vi "Master_WriteToDigOut.vi"(8 "error in":errorcluster, 9 "FPGA VI Reference In":refnum<k20>, 10 "Actuators in":T1) -> (0 "error out":errorcluster, 1 "FPGA VI Reference Out":refnum<k20>, 2 "Actuators out":T1)   [LabVIEW 2017]
uses:
  TypeDef_DigitalOuts.ctl
  <vilib>/Utility/error.llb/Error Cluster From Error Code.vi
  <vilib>/rvi/errors/niLvFpgaAdjustHostInterfaceError.vi
  <vilib>/rvi/interface/nirviReadWriteControl/nirviReadWriteControl.xnode
  NiFpgaLv.dll
  <vilib>/rvi/interface/Simulation/niFpgaSimulationCallBeginRW.vi
panel:
  out "Actual out":T1
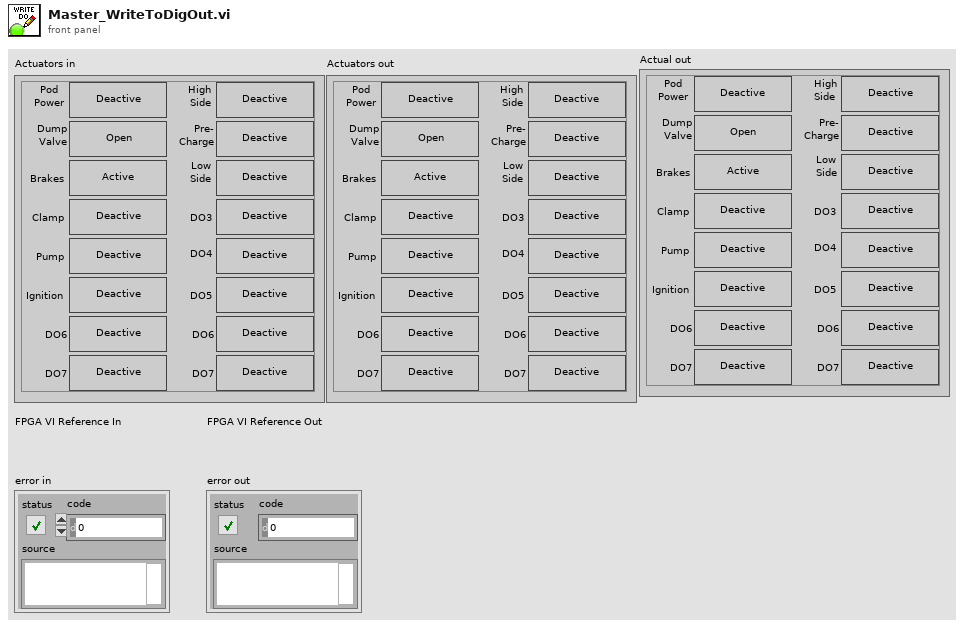
[diagram p1: front panel]
types:
  T1 = typedef "TypeDef_DigitalOuts.ctl" = cluster{"Pod Power":bool, "Dump Valve":bool, "Brakes":bool, "Clamp":bool, "Pump":bool, "Ignition":bool, "DO6":bool, "DO7":bool, "HighSide":bool, "Precharge":bool, "LowSide":bool, "DO3":bool, "DO4":bool, "DO5":bool, "DO62":bool, "DO72":bool}
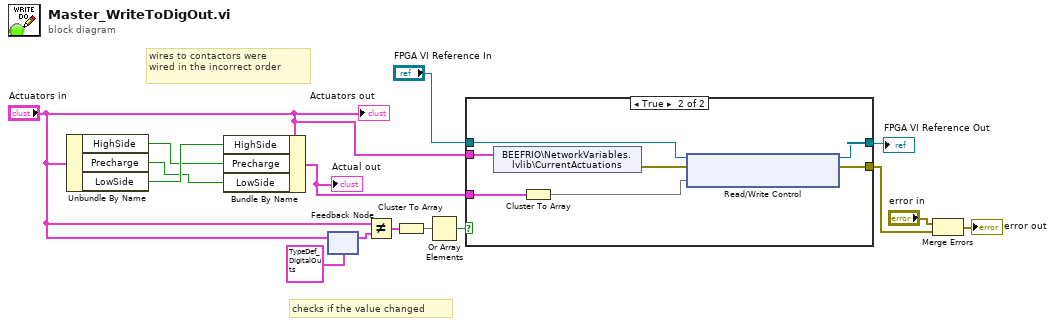
[diagram p0: block diagram]
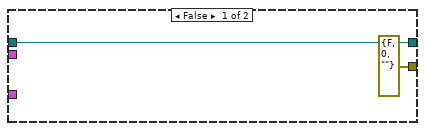
[diagram p2: hidden frame]
diagram:
  # "wires to contactors were\nwired in the incorrect order"
  # "checks if the value changed"
  n1 = Unbundle By Name("Actuators in") -> ("HighSide"=w2:bool, "Precharge"=w1:bool, "LowSide"=w3:bool)
  n2 = Bundle By Name(cluster="Actuators in", "HighSide"=w3, "Precharge"=w2, "LowSide"=w1) -> (w5:T1)
  "Actual out" <- w5
  n3 = feedback-in #1("Actuators in") -> ()
  n4 = feedback #1(T1 {"Pod Power"=FALSE, "Dump Valve"=FALSE, "Brakes"=FALSE, "Clamp"=FALSE, "Pump"=FALSE, "Ignition"=FALSE, "DO6"=FALSE, "DO7"=FALSE, "HighSide"=FALSE, "Precharge"=FALSE, "LowSide"=FALSE, "DO3"=FALSE, "DO4"=FALSE, "DO5"=FALSE, "DO62"=FALSE, "DO72"=FALSE} ("Actuators in")) -> (w15:T1)
  n5 = Not Equal?(x="Actuators in", y=w15) -> (x != y?=w12:T1)
  n6 = Cluster To Array(cluster=w12) -> (array=w11:bool[])
  n7 = Or Array Elements(Boolean array=w11) -> (logical OR=w14:bool)
  n8 = case shown="True" w14 {
    tunnel: [errorcluster {"status"=FALSE, "code"=0, "source"=""} ("error out") w24] -> w7
    tunnel: w5 -> [_ w18]
    tunnel: "FPGA VI Reference In" -> [w17 w22]
    tunnel: [w17 w23] -> w9
    tunnel: "Actuators in" -> [_ w19]
    frame False {
    }
    frame True {
      n9 = shared-variable "BEEFRIO\\NetworkVariables.lvlib\\CurrentActuations"(w19) -> (error out=w21:errorcluster)  [unwired: 1 in]
      n10 = Cluster To Array(cluster=w18) -> (array=w20:bool[])
      n11 = xnode "Read/Write Control"("FPGA VI Reference In"=w22, "error in"=w21, "Digital Control Outputs"=w20) -> ("FPGA VI Reference Out"=w23:refnum<k20>, "error out"=w24:errorcluster)
    }
  }
  "FPGA VI Reference Out" <- w9
  n12 = Merge Errors("error in", w7) -> (→"error out":errorcluster)
  "Actuators out" <- "Actuators in"
